vi "P1.vi"() -> ()   [LabVIEW 2020]
panel:
  out "Meter":dbl(knob) scale=0.0..100.0
  in  "Slide":dbl(slide) scale=0.0..100.0
  in  "Numeric":dbl
  out "Thermometer":dbl(slide) scale=0.0..100.0
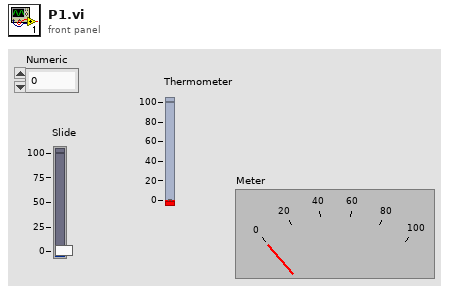
[diagram p1: front panel]
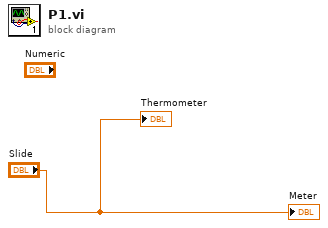
[diagram p0: block diagram]
diagram:
  "Thermometer" <- "Slide"
  "Meter" <- "Slide"
